vi "IT8800-Release.vi"(8 "error in":errorcluster, 11 "IT8800 Setting In":T1={"VISA Resource Name"="", "Baud Rate"=19200, "Stop Bits"=20, "Wait For Read(ms)"=0} {"Stop Bits" items=["1.0"=10, "2.0"=20]; "Baud Rate" items=["2400"=2400, "4800"=4800, "9600"=9600, "19200"=19200]}) -> (0 "error out":errorcluster)   [LabVIEW 2018]
uses:
  Data Def/IT8800-Setting.ctl
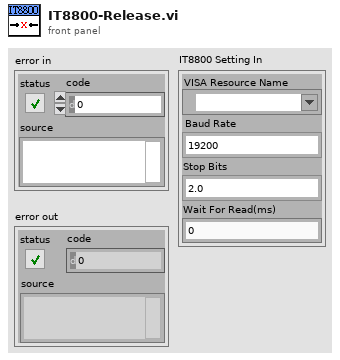
[diagram p1: front panel]
types:
  T1 = typedef "IT8800-Setting.ctl" = cluster{"VISA Resource Name":refnum<visa-resource-name>, "Baud Rate":u32, "Stop Bits":u16, "Wait For Read(ms)":u32}
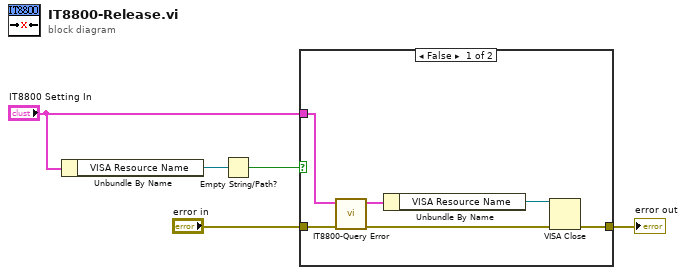
[diagram p0: block diagram]
diagram:
  n1 = Unbundle By Name("IT8800 Setting In") -> ("VISA Resource Name"=w2:refnum<visa-resource-name>)
  n2 = Empty String/Path?(string/path=w2) -> (empty?=w3:bool)
  n3 = case shown="False" w3 {
    tunnel: [w10 w12] -> w5
    tunnel: "error in" -> [w9 w12]
    tunnel: "IT8800 Setting In" -> [w8 _]
    frame False {
      n4 = call "IT8800-Query Error.vi"("error in"=w9, "IT8800 Setting In In"=w8) -> ("error out"=w11:errorcluster, "IT8800 Setting In Out"=w7:T1)  [unwired: 8 in]
      n5 = Unbundle By Name(w7) -> ("VISA Resource Name"=w6:refnum<visa-resource-name>)
      n6 = VISA Close(VISA resource name=w6, error in (no error)=w11) -> (error out=w10:errorcluster)
    }
    frame True {
    }
  }
  "error out" <- w5
